vi "AC_DC.vi"(0 "VisaCluster":T1, 7 "AC_DC":bool, 11 "error in (no error)":errorcluster) -> (4 "VisaCluster":T1, 6 "AC_DC  2":bool, 8 "Answer":string, 10 "Display":string, 15 "error out":errorcluster)   [LabVIEW 2014, in "FH 55.lvlib"]
doc: "This VI switchs between the AC-Modus and DC-Modus.\n\nDas VI AC_DC wechselt zwischen der Messung von Wechselfeldern (AC, periodisch alternierenden Magnetfeldern) und Gleichfeldern (DC, statischen Magnetfeldern)."
uses:
  FH 55.lvlib
  TypeDef/VisaCluster.ctl
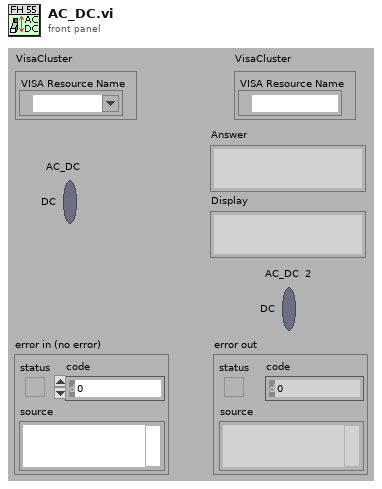
[diagram p1: front panel]
types:
  T1 = typedef "FH 55.lvlib/VisaCluster.ctl" = cluster{"VISA Resource Name":refnum<visa-resource-name>}
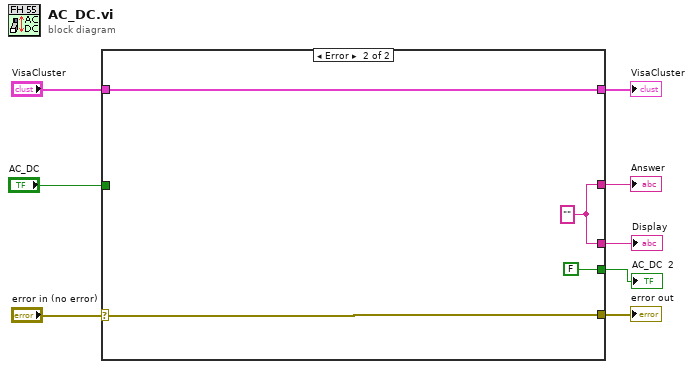
[diagram p0: block diagram]
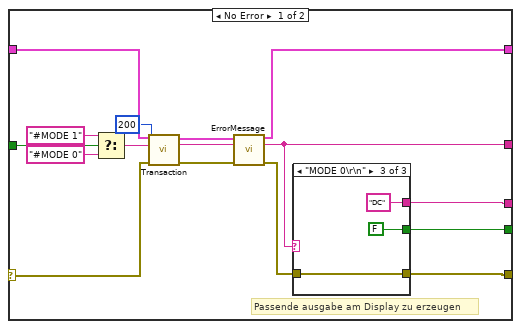
[diagram p2: hidden frame]
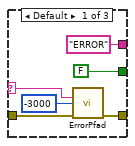
[diagram p3: hidden frame]
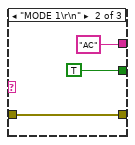
[diagram p4: hidden frame]
diagram:
  n1 = case shown="Error" "error in (no error)" {
    selector: "error in (no error)" -> [w18 w39]
    tunnel: "VisaCluster" -> [w20 w40]
    tunnel: "AC_DC" -> [w24 _]
    tunnel: [w21 w40] -> w4
    tunnel: [w11 w39] -> w6
    tunnel: [w13 w38] -> w5
    tunnel: [w14 w38] -> w2
    tunnel: [w9 FALSE] -> w1
    frame No Error {
      # "Passende ausgabe am Display zu erzeugen"
      n2 = Select(t="#MODE 1", s=w24, f="#MODE 0") -> (s? t:f=w19:string)
      n3 = call "Transaction.vi"("VisaCluster"=w20, "Command"=w19, "Time (150) ms"=u32 200, "error in (no error)"=w18) -> ("VisaCluster"=w15:T1, "Answer"=w16:string, "error out"=w17:errorcluster)  [unwired: 8 in, 1 out]
      n4 = call "ErrorMessage.vi"("VisaCluster"=w15, "Message In"=w16, "error in (no error)"=w17) -> ("VisaCluster"=w21:T1, "Message Out"=w13:string, "error out"=w12:errorcluster)  [unwired: 10 in]
      n5 = case shown="\"MODE 0\\r\\n\"" w13 {
        selector: w13 -> [w28 _ _]
        tunnel: ["ERROR" "AC" "DC"] -> w14
        tunnel: w12 -> [w29 w32 w35]
        tunnel: [w26 w32 w35] -> w11
        tunnel: [FALSE TRUE FALSE] -> w9
        frame Default {
          n6 = call "ErrorPfad.vi"("Message In"=w28, "Numeric"=-3000, "error in (no error)"=w29) -> ("error out"=w26:errorcluster)  [unwired: 11 in, 1 out]
        }
        frame "MODE 1\r\n" {
        }
        frame "MODE 0\r\n" {
        }
      }
    }
    frame Error {
      w38 = ""
    }
  }
  "error out" <- w6
  "Answer" <- w5
  "VisaCluster" <- w4
  "Display" <- w2
  "AC_DC  2" <- w1
